vi "getTimeStamps.vi"(8 "error in (no error)":errorcluster, 11 "RampEvent in":refnum<class "RampEvent.lvclass">) -> (0 "error out":errorcluster, 2 "timeStamps":dbl[](array[numeric]), 3 "RampEvent out":refnum<class "RampEvent.lvclass">)   [LabVIEW 2011, in "Tools.lvlib" / "Scripting.lvlib" / "RampEvent.lvclass"]
uses:
  RampEvent.lvclass
  ScriptEvent.lvclass
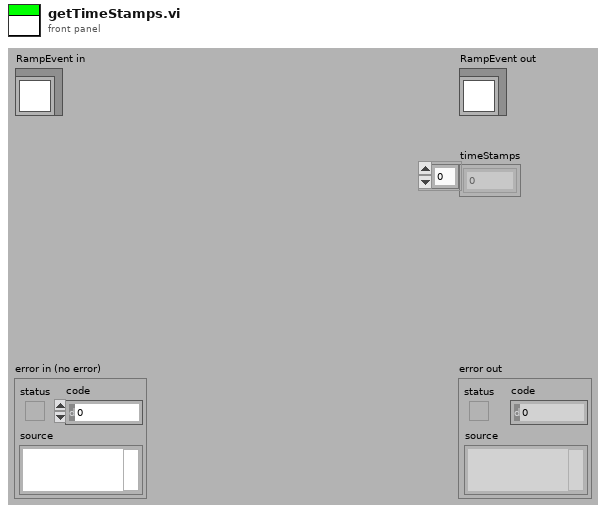
[diagram p1: front panel]
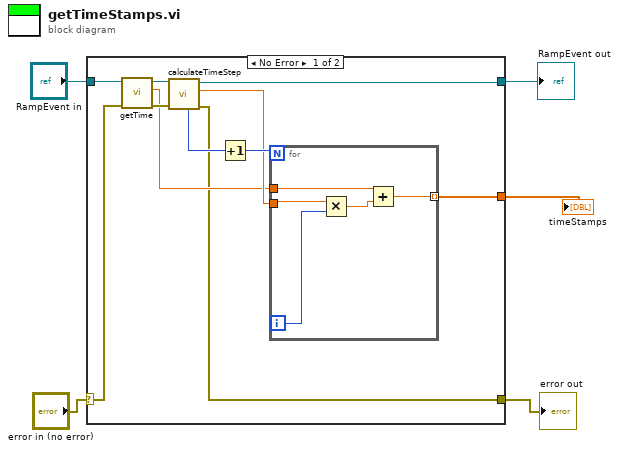
[diagram p0: block diagram]
diagram:
  n1 = case shown="No Error" "error in (no error)" {
    selector: "error in (no error)" -> [w13 w22]
    tunnel: [w7 w22] -> w4
    tunnel: "RampEvent in" -> [w14 w23]
    tunnel: [w8 w23] -> w2
    tunnel: [w6 _] -> w1
    frame No Error {
      n2 = call "getTime.vi"("error in (no error)"=w13, "ScriptEvent.lvclass in"=w14) -> ("error out"=w15:errorcluster, "time"=w9:dbl, "ScriptEvent.lvclass out"=w16:refnum<class "RampEvent.lvclass">)  [unwired: 7 in]
      n3 = call "calculateTimeStep.vi"("error in (no error)"=w15, "RampEvent in"=w16) -> ("error out"=w7:errorcluster, "timeStep"=w10:dbl, "RampEvent out"=w8:refnum<class "RampEvent.lvclass">, "number of Steps"=w12:i32)  [unwired: 5 in, 1 out]
      n4 = Increment(x=w12) -> (x+1=w11:i32)
      n5 = for {
        N: w11 -> [_]
        tunnel: w10 -> [w20]
        tunnel: w9 -> [w21]
        tunnel: [w17] -> w6 mode=indexing
        i -> [w18]
        n6 = Multiply(x=w20, y=w18) -> (x*y=w19:dbl)
        n7 = Add(x=w21, y=w19) -> (x+y=w17:dbl)
      }
    }
    frame Error {
    }
  }
  "error out" <- w4
  "RampEvent out" <- w2
  "timeStamps" <- w1
